vi "tqjcgy.vi"(0 "object in":refnum<class "212format_work.lvclass">, 1 "in":T1, 5 "error in (no error)":errorcluster) -> (14 "object out":refnum<class "212format_work.lvclass">, 15 "out":T2, 19 "error out":errorcluster)   [LabVIEW 2016, in "212format_work.lvclass"]
uses:
  212format_work.lvclass
  212format_work.lvclass/212format_work.ctl
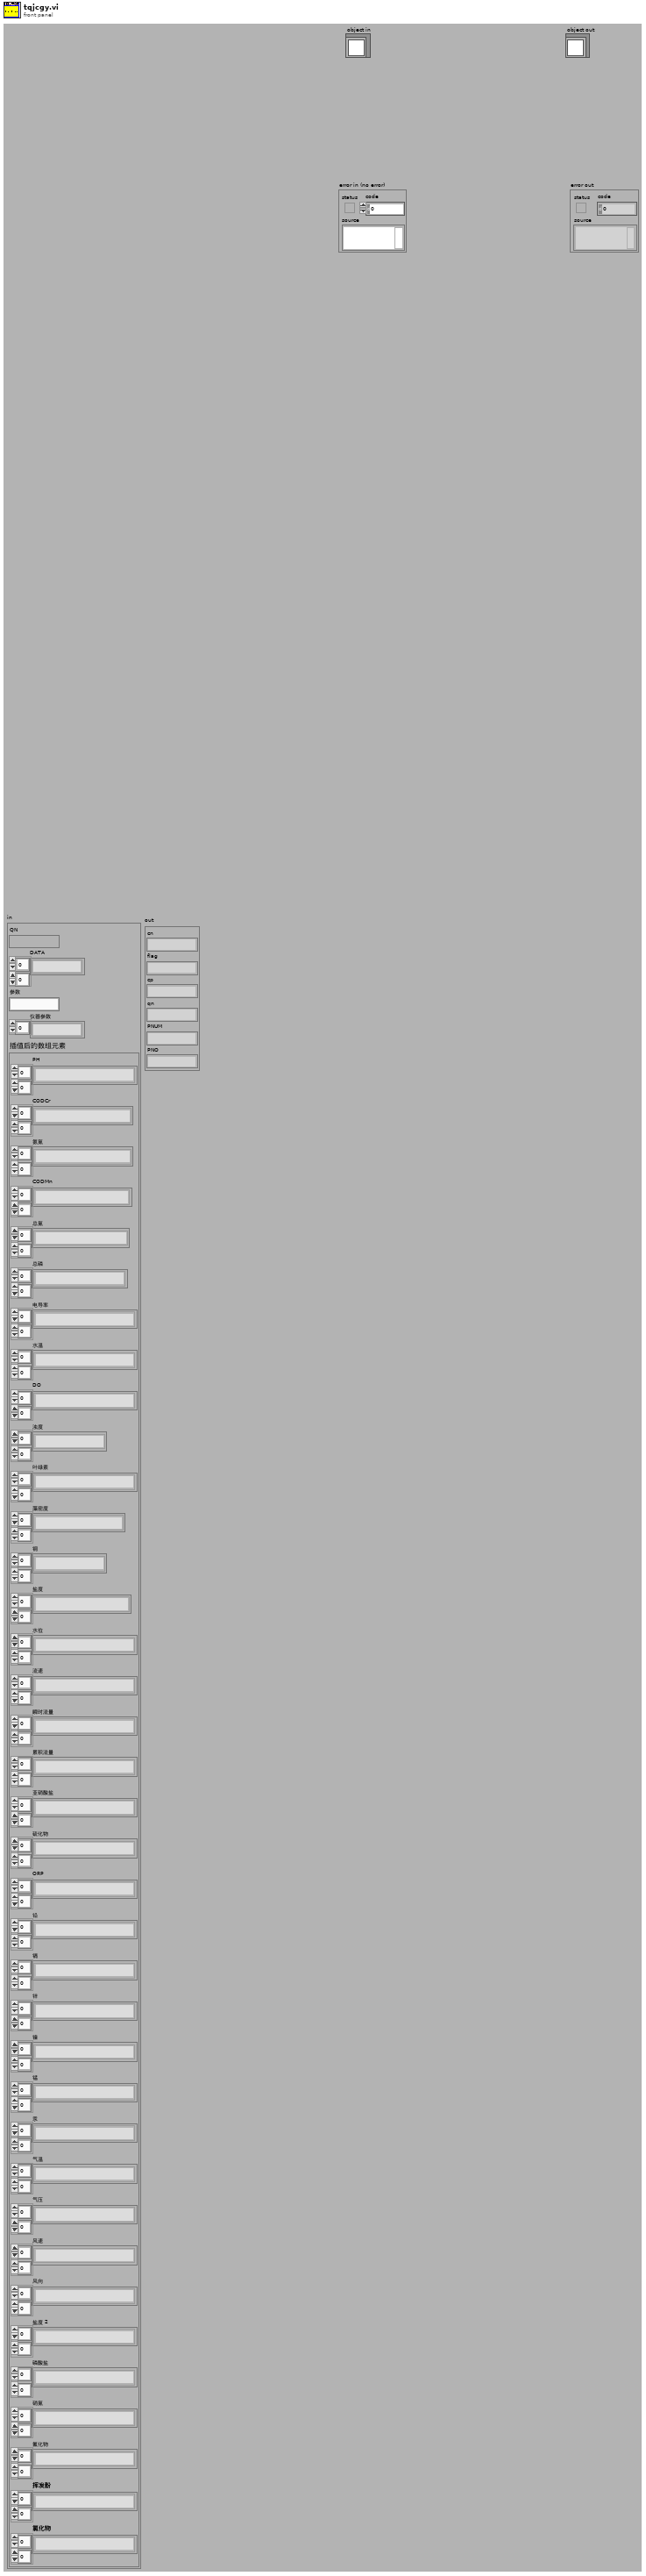
[diagram p1: front panel]
types:
  T1 = cluster{"QN":string, "DATA":string[][], "参数":string, "仪器参数":string[], "插值后的数组元素":cluster{"PH":string[][], "CODCr":string[][], "氨氮":string[][], "CODMn":string[][], "总氮":string[][], "总磷":string[][], "电导率":string[][], "水温":string[][], "DO":string[][], "浊度":string[][], "叶绿素":string[][], "藻密度":string[][], "铜":string[][], "盐度":string[][], "水位":string[][], "流速":string[][], "瞬时流量":string[][], "累积流量":string[][], "亚硝酸盐":string[][], "硫化物":string[][], "ORP":string[][], "铅":string[][], "镉":string[][], "锌":string[][], "镍":string[][], "锰":string[][], "汞":string[][], "气温":string[][], "气压":string[][], "风速":string[][], "风向":string[][], "盐度 2":string[][], "磷酸盐":string[][], "硝氮":string[][], "氟化物":string[][], "挥发酚":string[][], "氯化物":string[][]}}
  T2 = cluster{"cn":string, "flag":string, "cp":string, "qn":string, "PNUM":string, "PNO":string}
  T3 = enum16{"formattime", "formatminute", "formathour"}
  T4 = enum16{"小时数据", "实时数据", "平行样测试", "集成干预测试", "加标回收测试", "核查数据", "空白零点跨度数据", "提取小时数据", "提取实时数据", "操作日志", "仪器参数", "3090仪器参数", "提取仪器参数", "报警信息"}
  T5 = typedef "212format_work.lvclass/interdata控件.ctl" = cluster{"数据发送协议":enum16{"2005-212协议", "2017-212协议"}, "枚举":enum16{"返回请求应答", "上传数据", "返回执行结果"}, "系统编码ST":string, "主动上报数据中":bool, "数据组合发送":bool, "地表水/污染源":bool, "应用环境":enum16{"STD", "GB212"}}
  T6 = typedef "212format_work.lvclass/data控件.ctl" = cluster{"选择发送的参数":string, "插值后的数组元素":cluster{"PH":string[][], "CODCr":string[][], "氨氮":string[][], "CODMn":string[][], "总氮":string[][], "总磷":string[][], "电导率":string[][], "水温":string[][], "DO":string[][], "浊度":string[][], "叶绿素":string[][], "藻密度":string[][], "铜":string[][], "盐度":string[][], "水位":string[][], "流速":string[][], "瞬时流量":string[][], "累积流量":string[][], "亚硝酸盐":string[][], "硫化物":string[][], "ORP":string[][], "铅":string[][], "镉":string[][], "锌":string[][], "镍":string[][], "锰":string[][], "汞":string[][], "气温":string[][], "气压":string[][], "风速":string[][], "风向":string[][], "盐度 2":string[][], "磷酸盐":string[][], "硝氮":string[][], "氟化物":string[][], "挥发酚":string[][], "氯化物":string[][]}, "register values":u16[], "columns输出":string[], "环境参数":string[][], "仪器编码":string, "实时数据发送间隔":u32, "实时数据参数":string, "参数系数簇":cluster{"CODMn":dbl, "CODCr":dbl, "DO":dbl, "铜":dbl, "PH":dbl, "氨氮":dbl, "比电导率":dbl, "水温":dbl, "COD":dbl, "浊度":dbl, "总氮":dbl, "总磷":dbl, "叶绿素a":dbl, "藻密度":dbl, "水位":dbl, "流速":dbl, "瞬时流量":dbl, "累积流量":dbl, "亚硝酸盐":dbl, "硫化物":dbl, "ORP":dbl, "铅":dbl, "镉":dbl, "锌":dbl, "镍":dbl, "锰":dbl, "汞":dbl, "气温":dbl, "气压":dbl, "风速":dbl, "风向":dbl, "盐度":dbl, "磷酸盐":dbl, "硝氮":dbl, "氟化物":dbl, "挥发酚":dbl, "氯化物":dbl}, "因子编码簇":cluster{"CODMn":string, "CODCr":string, "DO":string, "铜":string, "PH":string, "氨氮":string, "比电导率":string, "水温":string, "COD":string, "浊度":string, "总氮":string, "总磷":string, "叶绿素a":string, "藻密度":string, "水位":string, "流速":string, "瞬时流量":string, "累积流量":string, "亚硝酸盐":string, "硫化物":string, "ORP":string, "铅":string, "镉":string, "锌":string, "镍":string, "锰":string, "汞":string, "气温":string, "气压":string, "风速":string, "风向":string, "盐度":string, "磷酸盐":string, "硝氮":string, "氟化物":string, "挥发酚":string, "氯化物":string}, "小时数据发送次数":i32, "读取试剂余量的值":u16[], "参数编码":string, "数据数组大小":i32, "总包数":i32, "当前包号":i32, "columns":string[], "剖面多参数":string[][], "分包标准":i32}
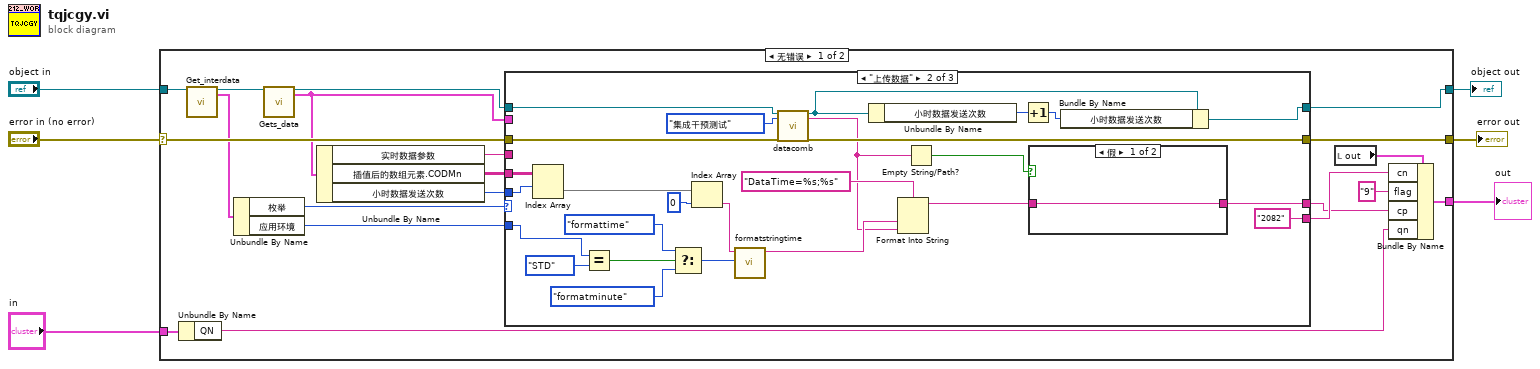
[diagram p0: block diagram]
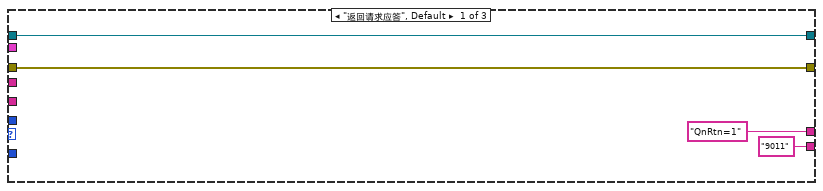
[diagram p2: hidden frame]
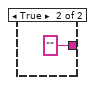
[diagram p3: hidden frame]
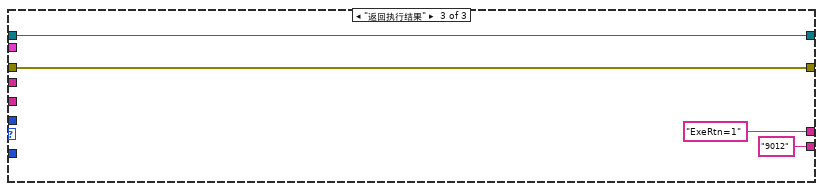
[diagram p4: hidden frame]
diagram:
  n1 = case shown="无错误" "error in (no error)" {
    selector: "error in (no error)" -> [w25 w64]
    tunnel: [w7 w64] -> w5
    tunnel: [w8 w63] -> w3
    tunnel: "object in" -> [w26 w63]
    tunnel: "in" -> [w24 _]
    tunnel: [w23 _] -> w1
    frame No Error {
      n2 = Unbundle By Name(w24) -> ("QN"=w18:string)
      n3 = call-dynamic "Get_interdata.vi"("object in"=w26) -> ("object out"=w15:refnum<class "212format_work.lvclass">, "interdata"=w17:T5)  [unwired: 16 in, 1 out]
      n4 = Unbundle By Name(w17) -> ("枚举"=w16:enum16{"返回请求应答", "上传数据", "返回执行结果"}, "应用环境"=w9:enum16{"STD", "GB212"})
      n5 = call-dynamic "Gets_data.vi"("object in"=w15) -> ("object out"=w13:refnum<class "212format_work.lvclass">, "data"=w10:T6)  [unwired: 16 in, 1 out]
      n6 = Unbundle By Name(w10) -> ("实时数据参数"=w14:string, "插值后的数组元素.CODMn"=w12:string[][], "小时数据发送次数"=w11:i32)
      n7 = case shown="\"上传数据\"" w16 {
        tunnel: ["9011" ("CN") "2082" ("CN") "9012" ("CN")] -> w21
        tunnel: ["QnRtn=1" w55 "ExeRtn=1"] -> w19
        tunnel: w14 -> [_ _ _]
        tunnel: w13 -> [w28 w56 w59]
        tunnel: [w28 w39 w59] -> w8
        tunnel: w25 -> [w27 w54 w60]
        tunnel: [w27 w53 w60] -> w7
        tunnel: w12 -> [_ w52 _]
        tunnel: w11 -> [_ w51 _]
        tunnel: w10 -> [_ _ _]
        tunnel: w9 -> [_ w36 _]
        frame "返回请求应答", Default {
        }
        frame "上传数据" {
          n8 = Index Array(array=w52, index (row)=w51) -> (element=w49:string[])  [unwired: 1 in]
          n9 = Equal?(x=w36, y=enum16{"STD", "GB212"}."STD") -> (x = y?=w34:bool)
          n10 = Select(t=T3."formattime" ("枚举"), s=w34, f=T3."formatminute" ("枚举")) -> (s? t:f=w31:T3)
          n11 = Index Array(array=w49, index=0 ("索引")) -> (element=w47:string)
          n12 = call "formatstringtime.vi"("枚举"=w31, "字符串"=w47) -> ("result string"=w44:string)  [unwired: 9 in]
          n13 = call-dynamic "datacomb.vi"("object in"=w56, "枚举"=T4."集成干预测试", "error in (no error)"=w54) -> ("object out"=w38:refnum<class "212format_work.lvclass">, "字符串"=w43:string, "error out"=w53:errorcluster)  [unwired: 14 in]
          n14 = Unbundle By Name(w38) -> ("小时数据发送次数"=w41:i32)
          n15 = Format Into String(format string="DataTime=%s;%s", w44, w43) -> (resulting string=w42:string)  [unwired: 2 in, 1 out]
          n16 = Empty String/Path?(string/path=w43) -> (empty?=w45:bool)
          n17 = Increment(x=w41) -> (x+1=w40:i32)
          n18 = case shown="假" w45 {
            tunnel: [w57 ""] -> w55
            tunnel: w42 -> [w57 _]
            frame False {
            }
            frame True {
            }
          }
          n19 = Bundle By Name(cluster=w38, "小时数据发送次数"=w40) -> (w39:refnum<class "212format_work.lvclass">)
        }
        frame "返回执行结果" {
        }
      }
      n20 = local read "out"() -> (w22:T2)
      n21 = Bundle By Name(cluster=w22, "cn"=w21, "flag"="9" ("ST"), "cp"=w19, "qn"=w18) -> (w23:T2)
    }
    frame Error {
    }
  }
  "error out" <- w5
  "object out" <- w3
  "out" <- w1
